vi "Simulated data.vi"(8 "error in (no error)":errorcluster, 9 "Sim multiplier":dbl, 10 "Waveforms array in":waveform(dbl)[](array[waveform]), 11 "Sim":bool) -> (3 "waveform":waveform(dbl))   [LabVIEW 2017]
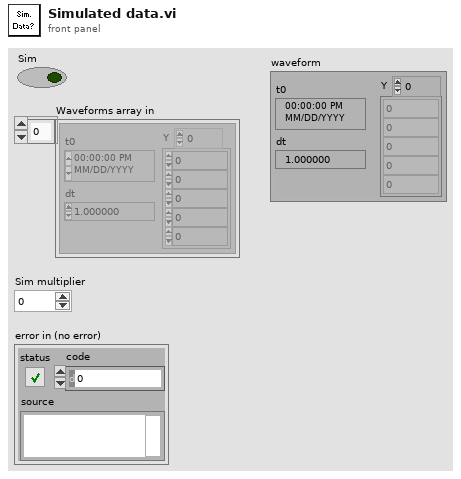
[diagram p1: front panel]
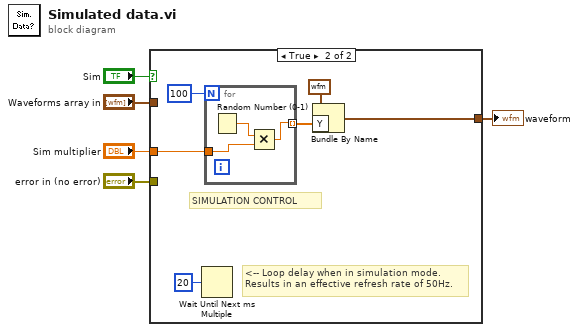
[diagram p0: block diagram]
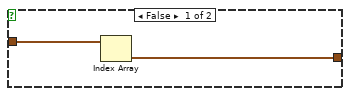
[diagram p2: hidden frame]
diagram:
  n1 = case shown="True" "Sim" {
    tunnel: [w6 w13] -> w3
    tunnel: "Waveforms array in" -> [w7 _]
    tunnel: "error in (no error)" -> [_ _]
    tunnel: "Sim multiplier" -> [_ w9]
    frame False {
      n2 = Index Array(array=w7) -> (element=w6:waveform(dbl))  [unwired: 1 in]
    }
    frame True {
      # "<-- Loop delay when in simulation mode.\nResults in an effective refresh rate of 50Hz."
      # "SIMULATION CONTROL"
      n3 = Wait Until Next ms Multiple(millisecond multiple=u32 20) -> ()  [unwired: 1 out]
      n4 = for {
        N: 100 -> [_]
        tunnel: [w15] -> w11 mode=indexing
        tunnel: w9 -> [w14]
        n5 = Random Number (0-1)() -> (number: 0 to 1=w16:dbl)
        n6 = Multiply(x=w16, y=w14) -> (x*y=w15:dbl)
      }
      n7 = Bundle By Name(cluster=waveform(dbl) {"t0"=timestamp(0 s since 1904-01-01), "dt"=1.0, "Y"=[]} ("waveform"), "Y"=w11) -> (w13:waveform(dbl))
    }
  }
  "waveform" <- w3
